vi "Operation UI.vi"(0 "Add in":refnum<class "Add.lvclass">, 5 "A":dbl, 7 "B":dbl, 9 "Calculate":bool, 11 "Error In":errorcluster, 12 "Stop":refnum<user-event>, 13 "Class Data":refnum<user-event>) -> (4 "Add out":refnum<class "Add.lvclass">, 6 "C":dbl, 15 "Error Out":errorcluster)   [LabVIEW 2023, in "Add.lvclass"]
doc: "The VI contains the addition operation UI that accepts two input numbers and performs addition operation and displays the output when user clicks calculate button"
uses:
  Add.lvclass
  C:/Users/Ancy.Augustin/Downloads/LVOOPS DVR/LVOOPS DVR/Classes/Arithemtic Operation/Arithemetic Operation.lvclass
  Arithemtic Operation/Arithemetic Operation.lvclass
  Typedef/User Event Operations.ctl
panel:
  # "ADDITION"
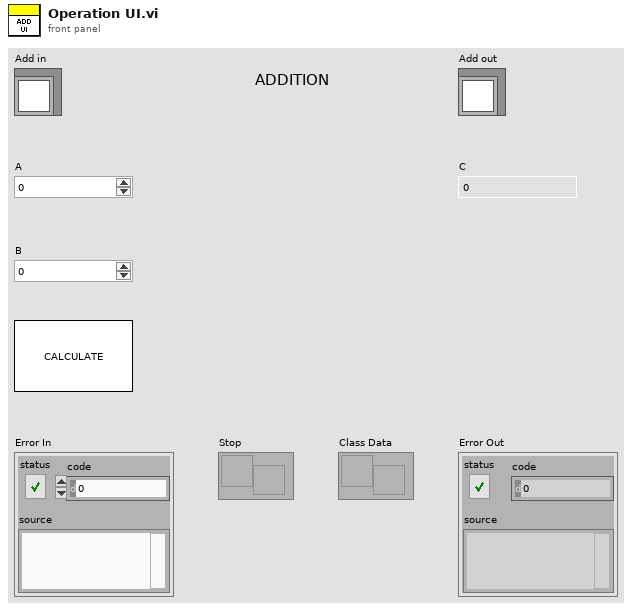
[diagram p1: front panel]
types:
  T1 = typedef "User Event Operations.ctl" = enum16{"Obtain", "Generate", "Release"}
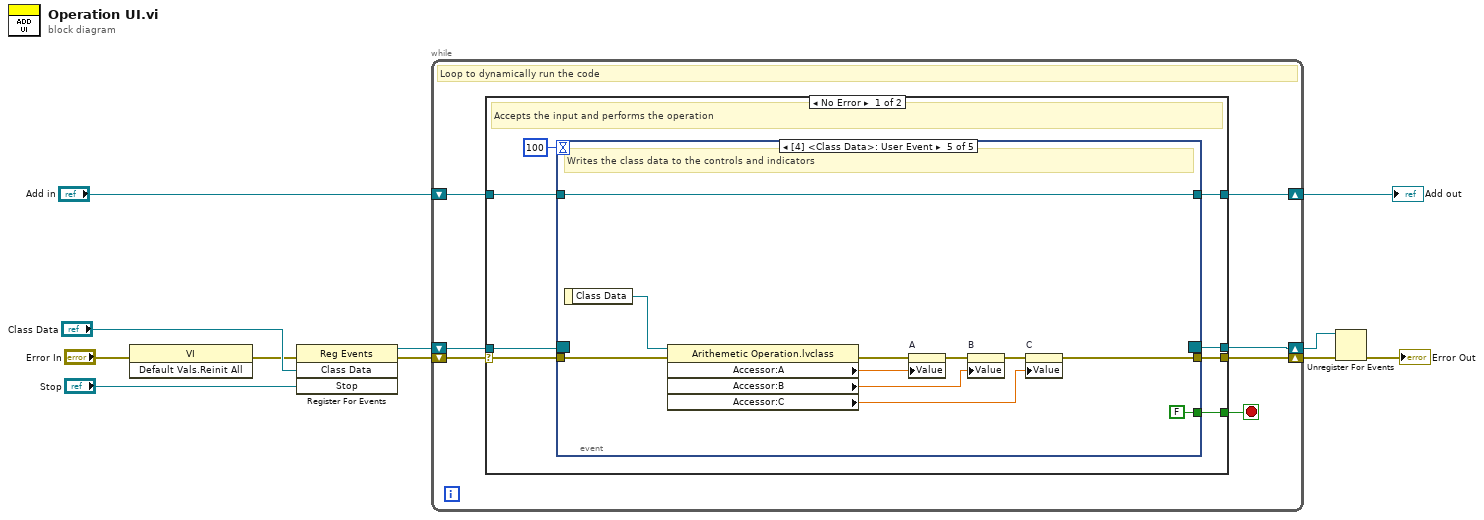
[diagram p0: block diagram]
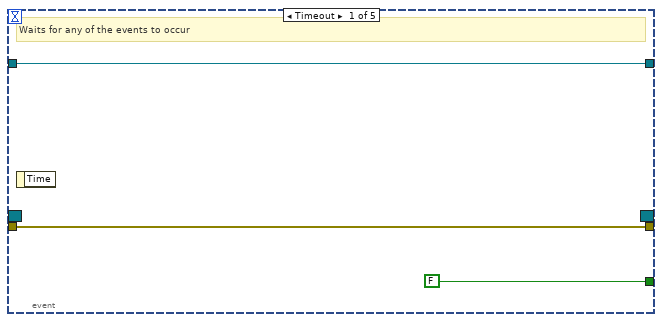
[diagram p2: hidden frame]
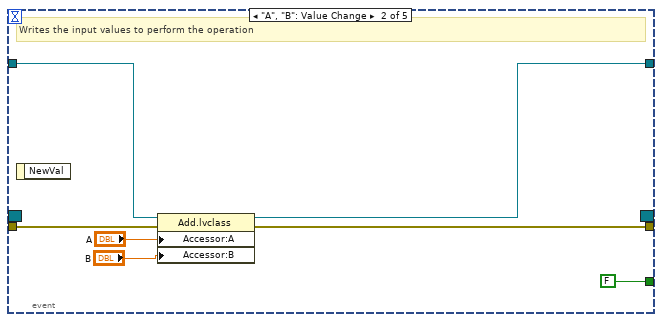
[diagram p3: hidden frame]
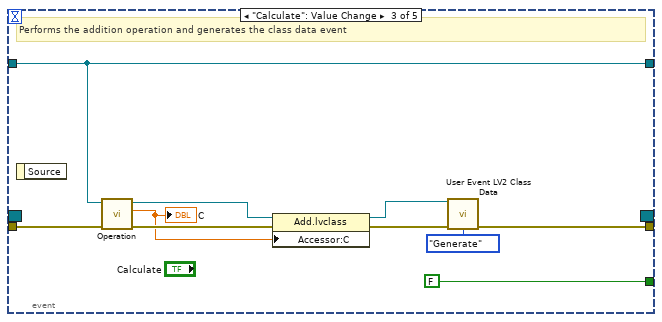
[diagram p4: hidden frame]
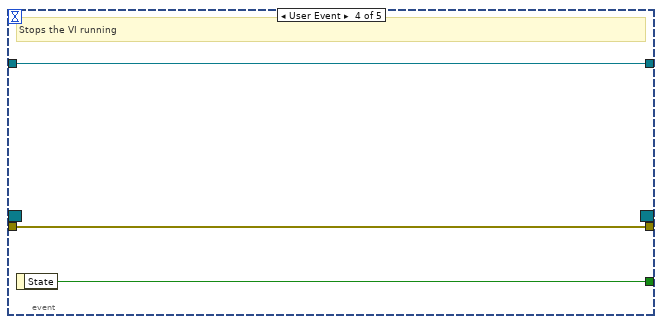
[diagram p5: hidden frame]
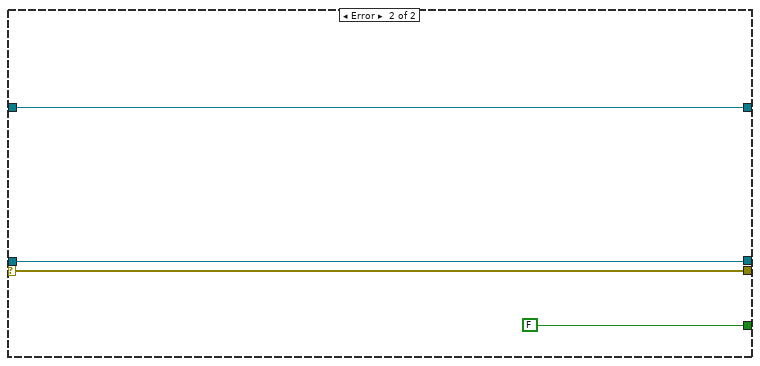
[diagram p6: hidden frame]
diagram:
  n1 = invoke class="VI" method="Default Vals.Reinit All"(error in="Error In") -> (error out=w1:errorcluster)  [unwired: 2 in, 2 out]
  n2 = register-events(error in=w1, "Class Data", "Stop") -> (reference out=w7:refnum<event-registration>, error out=w8:errorcluster)  [unwired: 1 in]
  n3 = while {
    shift-right: [w17] -> w11
    shift-left: w8 -> [w18]
    shift-right: [w15] -> w9
    shift-left: "Add in" -> [w16]
    shift-right: [w12] -> w4
    shift-left: w7 -> [w14]
    stop <- w13 stop-if-true
    # "Loop to dynamically run the code"
    n4 = case shown="No Error" w18 {
      selector: w18 -> [w24 w64]
      tunnel: [w23 w64] -> w17
      tunnel: [w25 w63] -> w15
      tunnel: w16 -> [w26 w63]
      tunnel: w14 -> [w21 w62]
      tunnel: [w20 w62] -> w12
      tunnel: [w19 FALSE] -> w13
      frame No Error {
        # "Accepts the input and performs the operation"
        n5 = event shown="[4] <Class Data>: User Event" {
          selector: w21 -> [_ _ _ _ _]
          dyn-events: [_ _ _ _ _] -> w20
          timeout: 100 -> [_ _ _ _ _]
          tunnel: [w29 w31 w42 w49 w60] -> w25
          tunnel: w26 -> [w29 w34 w42 w49 w60]
          tunnel: w24 -> [w28 w36 w46 w48 w59]
          tunnel: [w28 w35 w43 w48 w53] -> w23
          tunnel: [FALSE FALSE FALSE w47 FALSE] -> w19
          event Timeout {
            # "Waits for any of the events to occur"
            n6 = event-data() -> ()  [unwired: 1 in, 1 out]
          }
          event "A", "B": Value Change {
            # "Writes the input values to perform the operation"
            n7 = event-data() -> ()  [unwired: 1 in, 1 out]
            n8 = property class="Add.lvclass"(reference=w34, error in=w36, "Accessor:A"="A", "Accessor:B"="B") -> (reference out=w31:refnum<class "Add.lvclass">, error out=w35:errorcluster)
          }
          event "Calculate": Value Change {
            # "Performs the addition operation and generates the class data event"
            n9 = event-data() -> ()  [unwired: 1 in, 1 out]
            n10 = call-dynamic "Operation.vi"("Error In"=w46, "Add in"=w42) -> ("Error Out"=w45:errorcluster, "C"=w39:dbl, "Add out"=w40:refnum<class "Add.lvclass">)  [unwired: 7 in]
            "C" <- w39
            n11 = property class="Add.lvclass"(reference=w40, error in=w45, "Accessor:C"=w39) -> (reference out=w37:refnum<class "Add.lvclass">, error out=w41:errorcluster)
            n12 = call "User Event LV2 Class Data.vi"("Class Data"=w37, "Error In"=w41, "Operation"=User_Event_Operations."Generate") -> ("Error Out"=w43:errorcluster)  [unwired: 11 in, 1 out]
          }
          event User Event {
            # "Stops the VI running"
            n13 = event-data() -> ("State"=w47:bool)  [unwired: 1 in]
          }
          event User Event {
            # "Writes the class data to the controls and indicators"
            n14 = event-data() -> ("Class Data"=w56:refnum<class "Arithemetic Operation.lvclass">)  [unwired: 1 in]
            n15 = property class="Arithemetic Operation.lvclass"(reference=w56, error in=w59) -> (error out=w57:errorcluster, "Accessor:A"=w52:dbl, "Accessor:B"=w51:dbl, "Accessor:C"=w50:dbl)  [unwired: 1 out]
            n16 = property on="A" class="DigNum (strict)"(error in=w57, "Value"=w52) -> (error out=w54:errorcluster)  [unwired: 1 in, 1 out]
            n17 = property on="B" class="DigNum (strict)"(error in=w54, "Value"=w51) -> (error out=w55:errorcluster)  [unwired: 1 in, 1 out]
            n18 = property on="C" class="DigNum (strict)"(error in=w55, "Value"=w50) -> (error out=w53:errorcluster)  [unwired: 1 in, 1 out]
          }
        }
      }
      frame Error {
      }
    }
  }
  "Add out" <- w9
  n19 = Unregister For Events(event registration refnum=w4, error in=w11) -> (error out=→"Error Out":errorcluster)
